vi "Enable By Name.vi"(8 "error in (no error)":errorcluster, 9 "Enable Items":bool[](array[boolean]), 10 "Names":string[](array[string]), 11 "Selector in":refnum<class "Selector.lvclass">) -> (0 "error out":errorcluster, 3 "Selector out":refnum<class "Selector.lvclass">)   [LabVIEW 2019, in "Selector.lvclass"]
uses:
  Selector.lvclass
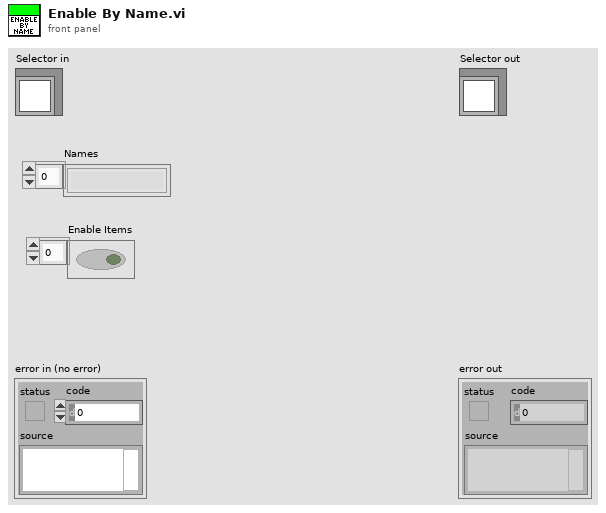
[diagram p1: front panel]
types:
  T1 = cluster{"Name":string, "Group":string, "Enabled":bool}[]
  T2 = cluster{"Name":string, "Group":string, "Enabled":bool}
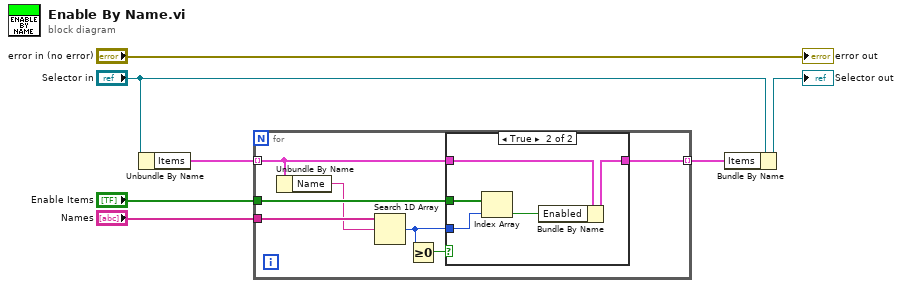
[diagram p0: block diagram]
diagram:
  n1 = Unbundle By Name("Selector in") -> ("Items"=w6:T1)
  n2 = for {
    tunnel: w6 -> [w14] mode=indexing
    tunnel: "Enable Items" -> [w9]
    tunnel: [w13] -> w3 mode=indexing
    tunnel: "Names" -> [w12]
    n3 = Unbundle By Name(w14) -> ("Name"=w8:string)
    n4 = Search 1D Array(1D array=w12, element=w8) -> (index of element=w10:i32)  [unwired: 1 in]
    n5 = Greater Or Equal To 0?(x=w10) -> (x >= 0?=w11:bool)
    n6 = case shown="True" w11 {
      tunnel: w10 -> [_ w19]
      tunnel: w9 -> [_ w20]
      tunnel: w14 -> [w15 w17]
      tunnel: [w15 w16] -> w13
      frame False {
      }
      frame True {
        n7 = Index Array(array=w20, index=w19) -> (element=w18:bool)
        n8 = Bundle By Name(cluster=w17, "Enabled"=w18) -> (w16:T2)
      }
    }
  }
  n9 = Bundle By Name(cluster="Selector in", "Items"=w3) -> (→"Selector out":refnum<class "Selector.lvclass">)
  "error out" <- "error in (no error)"
